vi "JTAG Read.vi"(7 "Function":T1(ring), 11 "error in (no error)":errorcluster) -> (6 "Manual Read":u8 format="%02x", 15 "error out":errorcluster)   [LabVIEW 2010]
panel:
  # "Manual Inputs"
  # "HIGH"
  # "LOW"
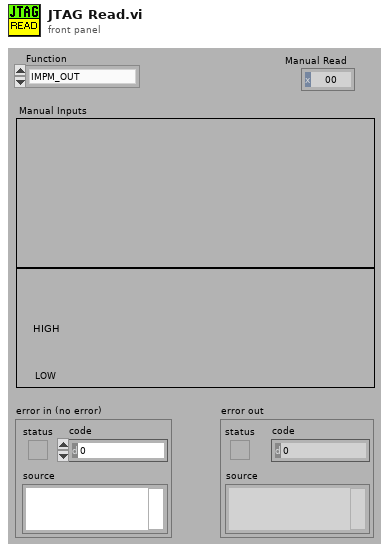
[diagram p1: front panel]
types:
  T1 = enum16{"IMPM_OUT", "PWR_ANA_OUT", "ACCEL_X", "ACCEL_Y", "ACCEL_Z", "CAL_RESIN", "CAL_RESOUT"}
  T2 = enum8{"PORT_OUT", "PORT_SEL", "PORT_RES_EN", "READ_PORT", "PORT_DIR", "SET_LCM", "PLUTO_WRITE_SINGLE", "PLUTO_READ_SINGLE", "PLUTO_WRITE_MASK", "STIM_POWER_UP", "STIM_POWER_DN", "SATURN_WRITE_SINGLE", "SATURN_READ_SINGLE", "SATURN_WRITE_BLOCK", "SATURN_READ_BLOCK", "SATURN_WRITE_MASK", "MICS_POWER_UP", "MICS_POWER_DN", "MICS_WRITE_SINGLE", "MICS_READ_SINGLE", "MICS_WRITE_BLOCK", "MICS_READ_BLOCK", "MICS_WRITE_MASK", "MEM_POWER_UP", "MEM_POWER_DN", "MEM_WRITE_SINGLE", "MEM_READ_SINGLE", "MEM_WRITE_BLOCK", "MEM_READ_BLOCK", "MEM_WRITE_MASK", "MEM_WRITE_SR", "MEM_READ_SR", "MEM_OPCODE", "INIT_VARIABLES", "DCO -> 1 MHz", "DCO -> 8 MHz", "START_STIM_CLK", "STOP_STIM_CLK", "PULSE_STIM_CLK", "PULSE_STIM_SCK", "SINGLE_ADC12", "SINGLE_ADC12_REPEAT", "MULTI_ADC12", "MULTI_ADC12_REPEAT", "Disable_ADC12", "READ_IO_VARIABLES"}
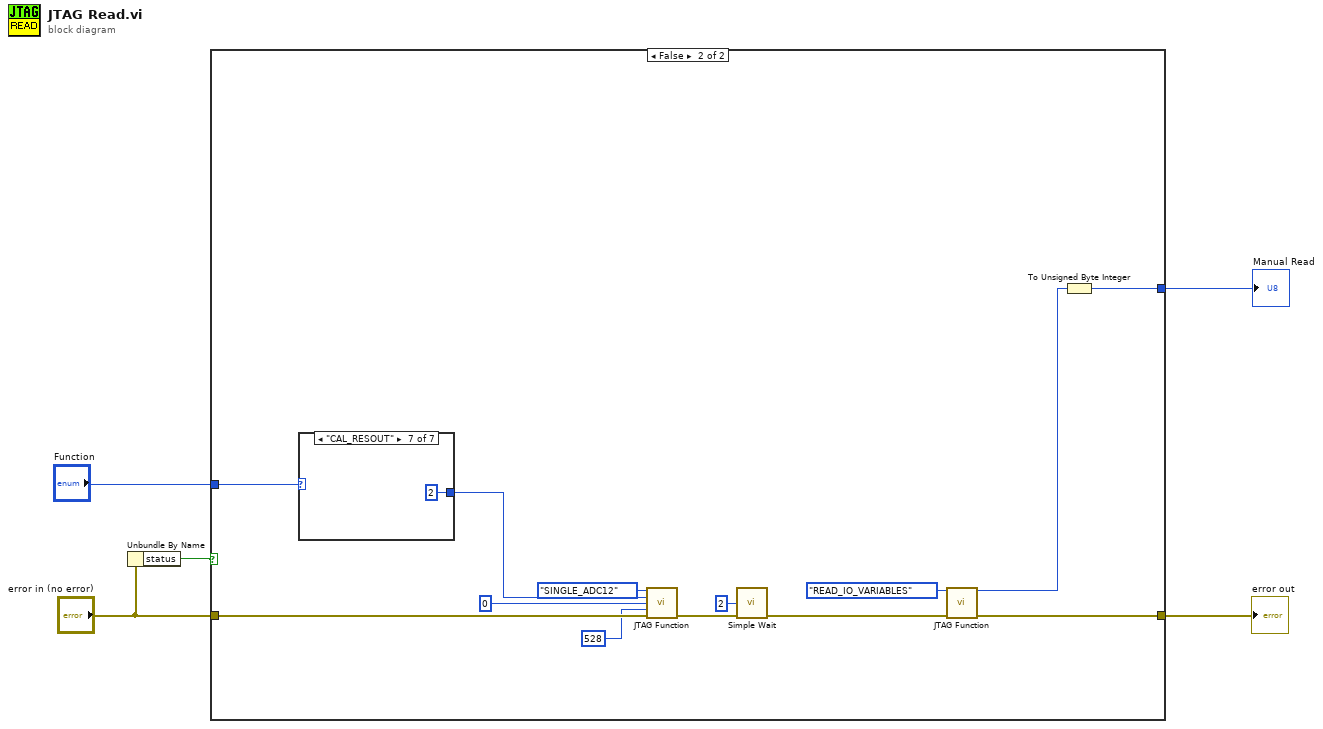
[diagram p0: block diagram]
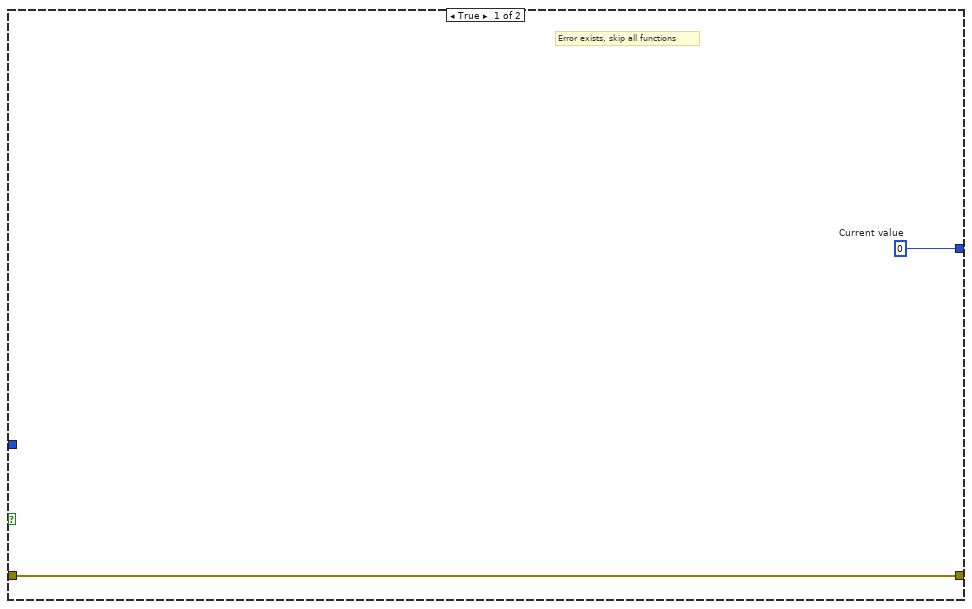
[diagram p2: hidden frame]
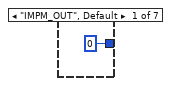
[diagram p3: hidden frame]
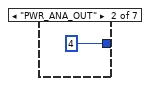
[diagram p4: hidden frame]
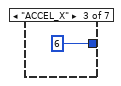
[diagram p5: hidden frame]
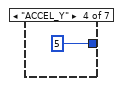
[diagram p6: hidden frame]
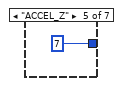
[diagram p7: hidden frame]
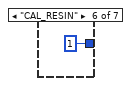
[diagram p8: hidden frame]
diagram:
  n1 = Unbundle By Name("error in (no error)") -> ("status"=w4:bool)
  n2 = case shown="False" w4 {
    tunnel: [w7 w18] -> w5
    tunnel: "error in (no error)" -> [w7 w20]
    tunnel: "Function" -> [_ w8]
    tunnel: [w6 w14] -> w2
    frame True {
      w6 = u8 0  # Current value
      # "Error exists, skip all functions"
    }
    frame False {
      n3 = case shown="\"CAL_RESOUT\"" w8 {
        tunnel: [u16 0 ("ARG 1") u16 4 ("ARG 1") u16 6 ("ARG 1") u16 5 ("ARG 1") u16 7 ("ARG 1") u16 1 ("ARG 1") u16 2 ("ARG 1")] -> w11
        frame "IMPM_OUT", Default {
        }
        frame "PWR_ANA_OUT" {
        }
        frame "ACCEL_X" {
        }
        frame "ACCEL_Y" {
        }
        frame "ACCEL_Z" {
        }
        frame "CAL_RESIN" {
        }
        frame "CAL_RESOUT" {
        }
      }
      n4 = call "JTAG Function.vi"("Enum"=T2."SINGLE_ADC12", "ARG 1"=w11, "ARG 2"=u16 0, "ARG 3"=u16 528, "error in (no error)"=w20) -> ("error out"=w19:errorcluster)  [unwired: 8 in, 2 out]
      n5 = call "Simple Wait.vi"("mS"=u32 2, "error in"=w19) -> ("error out"=w13:errorcluster)  [unwired: 12 in, 1 out]
      n6 = call "JTAG Function.vi"("Enum"=T2."READ_IO_VARIABLES", "error in (no error)"=w13) -> ("ARG 7"=w15:u16, "error out"=w18:errorcluster)  [unwired: 11 in, 1 out]
      n7 = To Unsigned Byte Integer(number=w15) -> (unsigned 8bit integer=w14:u8)
    }
  }
  "error out" <- w5
  "Manual Read" <- w2
